vi "Sensor Interface.vi"(8 "error in (no error)":errorcluster) -> (0 "error out":errorcluster)   [LabVIEW 2020]
doc: "Sensor Interface thread"
uses:
  Controls/Sensor Interface.ctl
  FGV/Controls/FGV_State.ctl
  Controls/Data_Initialize.ctl
  Database/Controls/Account Database.ctl
  Controls/Events_User.ctl
  SubVIs/Message Queue/Enqueue Message (Single).vi
  <vilib>/Utility/error.llb/Error Cluster From Error Code.vi
  <vilib>/ErrorRing/Error Ring.xnode
  SubVIs/User Event - Stop/User Event - Stop.lvlib
  SubVIs/Message Queue/Message Queue.lvlib
panel:
  in  "Sensor Interface":T1
  # "[Covers: UI4]"
  # "[Covers: UI1]"
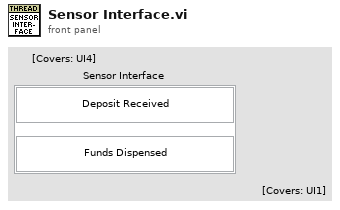
[diagram p1: front panel]
types:
  T1 = typedef "Sensor Interface.ctl" = cluster{"Deposit Received":bool, "Funds Dispensed":bool}
  T2 = enum32{"Invalid", "Standard", "Closed", "Hidden", "Minimized", "Maximized"}
  T3 = typedef "FGV_State.ctl" = enum16{"1 - OpenDatabase", "2 - Initialize Events", "3 - Initialize QMH", "4 - Close QMH", "5 - Close Events", "Read FGV", "Save Database", "Def"}
  T4 = typedef "FGV_Data.ctl" = cluster{"QMH":T5, "User Events":T6, "Database":T7[]}
  T5 = typedef "Message Queue.lvlib/All Message Queues.ctl" = cluster{"User Console":refnum<queue>, "Display Console":refnum<queue>, "Sensor Interface":refnum<queue>, "Process":refnum<queue>}
  T6 = typedef "Events_User.ctl" = cluster{"Stop User Console":refnum<user-event>, "Error User Console":refnum<user-event>, "Stop Sensor Interface ":refnum<user-event>, "Error Sensor Interface":refnum<user-event>}
  T7 = typedef "Account Database.ctl" = cluster{"Account Number":i32, "First Name":string, "Last Name":string, "Balance":dbl}
  T8 = typedef "Data_Initialize.ctl" = cluster{"Database":T7[], "User Events":T6}
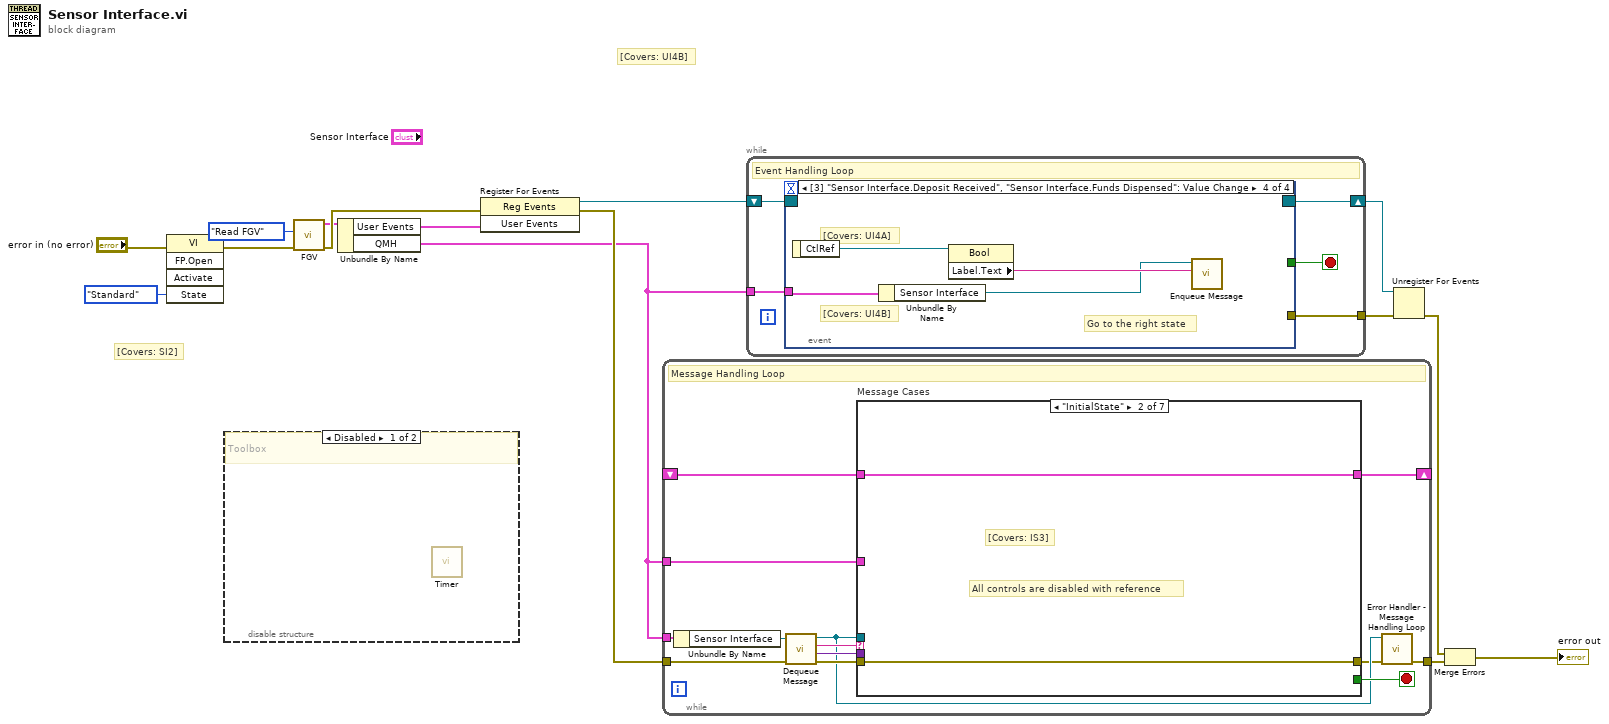
[diagram p0: block diagram]
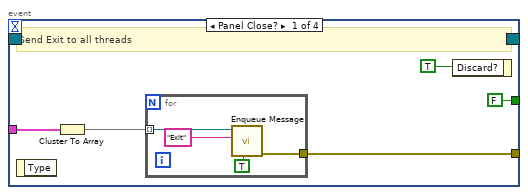
[diagram p3: hidden frame]
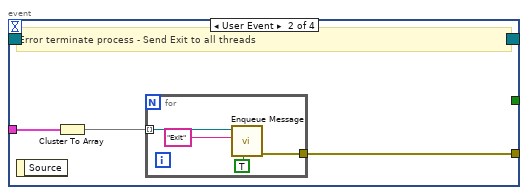
[diagram p4: hidden frame]
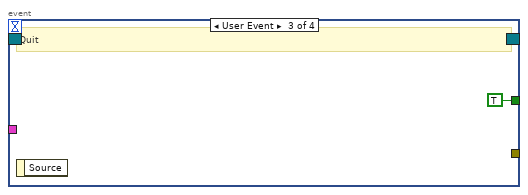
[diagram p5: hidden frame]
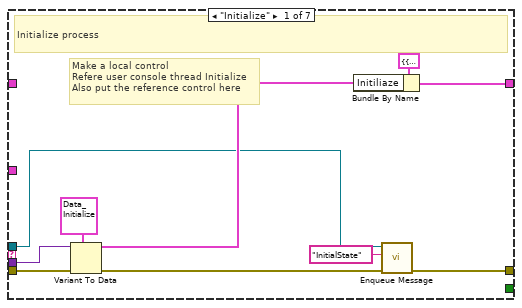
[diagram p6: hidden frame]
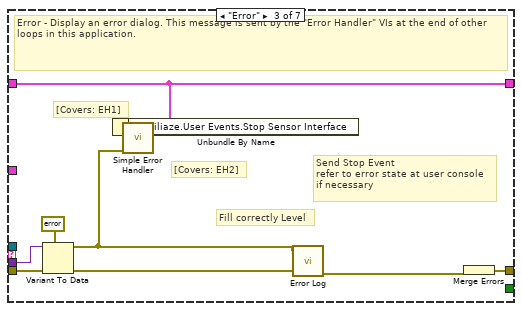
[diagram p7: hidden frame]
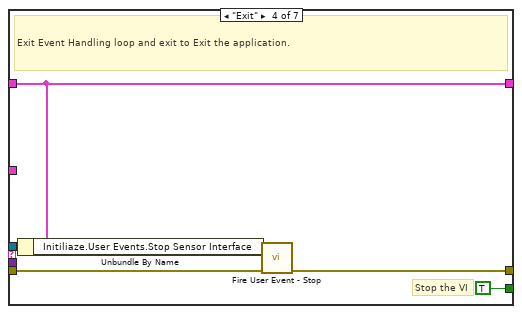
[diagram p8: hidden frame]
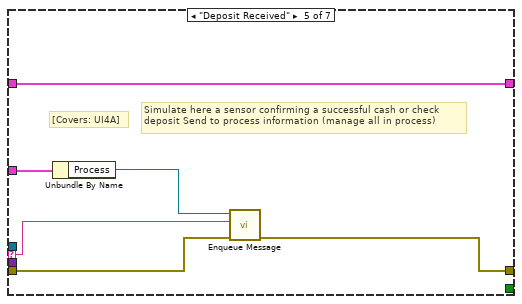
[diagram p9: hidden frame]
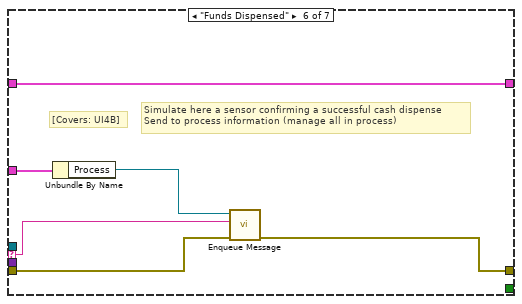
[diagram p10: hidden frame]
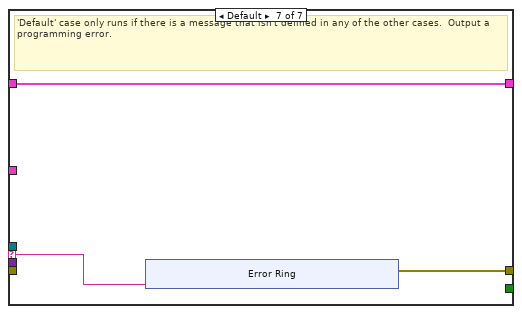
[diagram p11: hidden frame]
diagram:
  # "[Covers: UI4B]"
  # "[Covers: SI2]"
  n1 = invoke class="VI" method="FP.Open"(error in="error in (no error)", "State"=T2."Standard") -> (error out=w3:errorcluster)  [unwired: 3 in, 4 out]
  n2 = disable-structure shown="Disabled" {
    frame Disabled {
      # "Toolbox"
      n3 = call "Timer.vi"() -> ()  [unwired: 9 in, 3 out]
    }
    frame Enabled {
    }
  }
  n4 = call "FGV.vi"("error in (no error)"=w3, "FGV_State"=FGV_State."Read FGV") -> ("error out"=w13:errorcluster, "FGV 2"=w11:T4)  [unwired: 8 in]
  n5 = Unbundle By Name(w11) -> ("User Events"=w12:T6, "QMH"=w1:T5)
  n6 = register-events(error in=w13, w12) -> (reference out=w9:refnum<event-registration>, error out=w15:errorcluster)  [unwired: 1 in]
  n7 = while {
    tunnel: w1 -> [w18]
    shift-right: [w27] -> _
    shift-left: _ -> [w28]
    tunnel: w15 -> [w25]
    tunnel: [w20] -> w5
    tunnel: w1 -> [w16]
    stop <- w26 stop-if-true
    # "Message Handling Loop"
    n8 = Unbundle By Name(w18) -> ("Sensor Interface"=w17:refnum<queue>)
    n9 = call "Dequeue Message.vi"("error in (no error)"=w25, "Message Queue"=w17) -> ("error out"=w24:errorcluster, "Message Data"=w22:variant, "Message"=w23:string, "dup Message Queue"=w21:refnum<queue>)  [unwired: 6 in]
    n10 = case "Message Cases" shown="\"InitialState\"" w23 {
      selector: w23 -> [_ _ _ _ w56 w62 w66]
      tunnel: w21 -> [w32 _ _ _ _ _ _]
      tunnel: w24 -> [w36 w40 w48 w50 w55 w61 _]
      tunnel: [w30 w40 w45 w49 w54 w60 w67] -> w19
      tunnel: w28 -> [_ w39 w41 w52 w59 w65 w68]
      tunnel: [w38 w39 w41 w52 w59 w65 w68] -> w27
      tunnel: [_ _ _ TRUE _ _ _] -> w26
      tunnel: w22 -> [w33 _ w47 _ _ _ _]
      tunnel: w16 -> [_ _ _ _ w58 w64 _]
      frame "Initialize" {
        # "Make a local control\nRefere user console thread Initialize\nAlso put the reference control here"
        # "Initialize process"
        n11 = Variant To Data(error in=w36, type=T8 {"Database"=[], "User Events"={"Stop User Console"=refnum, "Error User Console"=refnum, "Stop Sensor Interface "=refnum, "Error Sensor Interface"=refnum}} ("Initiliaze"), Variant=w33) -> (data=w34:T8, error out=w31:errorcluster)
        n12 = Bundle By Name(cluster=cluster{"Initiliaze":T8} {"Initiliaze"={"Database"=[], "User Events"={"Stop User Console"=refnum, "Error User Console"=refnum, "Stop Sensor Interface "=refnum, "Error Sensor Interface"=refnum}}} ("Local Data"), "Initiliaze"=w34) -> (w38:cluster{"Initiliaze":T8})
        n13 = call-poly "Enqueue Message.vi"("error in (no error)"=w31, "Message"="InitialState", "Message Queue"=w32) -> ("error out"=w30:errorcluster)  [unwired: 7 in, 1 out]
      }
      frame "InitialState" {
        # "[Covers: IS3]"
        # "All controls are disabled with reference"
      }
      frame "Error" {
        # "Send Stop Event\nrefer to error state at user console \nif necessary"
        # "[Covers: EH2]"
        # "[Covers: EH1]"
        # "Fill correctly Level"
        # "Error - Display an error dialog. This message is sent by the \"Error Handler\" VIs at the end of other loops in this application."
        n14 = Variant To Data(error in=w48, type=errorcluster {"status"=FALSE, "code"=0, "source"=""} ("error constant"), Variant=w47) -> (data=w42:errorcluster, error out=w44:errorcluster)
        n15 = Unbundle By Name(w41) -> ()  [unwired: 1 out]
        n16 = call <vilib>:"Simple Error Handler.vi"("error in (no error)"=w42) -> ()  [unwired: 4 in, 5 out]
        n17 = call "Error Log.vi"("error in"=w44, "error happened"=w42) -> ("error out"=w43:errorcluster)  [unwired: 9 in]
        n18 = Merge Errors(w43) -> (w45:errorcluster)
      }
      frame "Exit" {
        # "Stop the VI"
        # "Exit Event Handling loop and exit to Exit the application."
        n19 = Unbundle By Name(w52) -> ("Initiliaze.User Events.Stop Sensor Interface"=w51:refnum<user-event>)
        n20 = call "Fire User Event - Stop.vi"("error in (no error)"=w50, "User Event - Stop"=w51) -> ("error out"=w49:errorcluster)  [unwired: 9 in]
      }
      frame "Deposit Received" {
        # "Simulate here a sensor confirming a successful cash or check\ndeposit Send to process information (manage all in process)"
        # "[Covers: UI4A]"
        n21 = Unbundle By Name(w58) -> ("Process"=w57:refnum<queue>)
        n22 = call-poly "Enqueue Message.vi"("error in (no error)"=w55, "Message"=w56, "Message Queue"=w57) -> ("error out"=w54:errorcluster)  [unwired: 7 in, 1 out]
      }
      frame "Funds Dispensed" {
        # "Simulate here a sensor confirming a successful cash dispense \nSend to process information (manage all in process)"
        # "[Covers: UI4B]"
        n23 = Unbundle By Name(w64) -> ("Process"=w63:refnum<queue>)
        n24 = call-poly "Enqueue Message.vi"("error in (no error)"=w61, "Message"=w62, "Message Queue"=w63) -> ("error out"=w60:errorcluster)  [unwired: 7 in, 1 out]
      }
      frame Default {
        # "'Default' case only runs if there is a message that isn't defined in any of the other cases.  Output a programming error."
        n25 = xnode "Error Ring"("parameter 0"=w66) -> ("error out"=w67:errorcluster)
      }
    }
    n26 = call "Error Handler - Message Handling Loop.vi"("error in (no error)"=w19, "Message Queue"=w21) -> ("dup error in"=w20:errorcluster)  [unwired: 8 in, 1 out]
  }
  n27 = while {
    tunnel: w1 -> [w80]
    shift-right: [w78] -> w7
    shift-left: w9 -> [w79]
    tunnel: [w76] -> w8
    stop <- w77 stop-if-true
    # "Event Handling Loop"
    n28 = event shown="[3] \"Sensor Interface.Deposit Received\", \"Sensor Interface.Funds Dispensed\": Value Change" {
      selector: w79 -> [_ _ _ _]
      dyn-events: [_ _ _ _] -> w78
      timeout: _ -> [_ _ _ _]
      tunnel: [FALSE ("Discard?") _ TRUE ("Discard?") _] -> w77
      tunnel: w80 -> [w84 w92 _ w98]
      tunnel: [w83 w91 _ _] -> w76
      event Panel Close? {
        # "Send Exit to all threads"
        n29 = event-data() -> ()  [unwired: 1 in, 1 out]
        n30 = Cluster To Array(cluster=w84) -> (array=w82:refnum<queue>[])
        n31 = for {
          tunnel: w82 -> [w89] mode=indexing
          tunnel: [w88] -> w83
          n32 = call-poly "Enqueue Message.vi"("Priority Message? (F)"=TRUE, "Message"="Exit", "Message Queue"=w89) -> ("error out"=w88:errorcluster)  [unwired: 7 in, 1 out]
        }
        n33 = event-data("Discard?"=TRUE) -> ()  [unwired: 1 in, 1 out]
      }
      event User Event {
        # "Error terminate process - Send Exit to all threads"
        n34 = event-data() -> ()  [unwired: 1 in, 1 out]
        n35 = Cluster To Array(cluster=w92) -> (array=w90:refnum<queue>[])
        n36 = for {
          tunnel: w90 -> [w96] mode=indexing
          tunnel: [w95] -> w91
          n37 = call-poly "Enqueue Message.vi"("Priority Message? (F)"=TRUE, "Message"="Exit", "Message Queue"=w96) -> ("error out"=w95:errorcluster)  [unwired: 7 in, 1 out]
        }
      }
      event User Event {
        # "Quit"
        n38 = event-data() -> ()  [unwired: 1 in, 1 out]
      }
      event Value Change {
        # "[Covers: UI4B]"
        # "Go to the right state"
        # "[Covers: UI4A]"
        n39 = event-data() -> ("CtlRef"=w99:refnum<vi>)  [unwired: 1 in]
        n40 = Unbundle By Name(w98) -> ("Sensor Interface"=w100:refnum<queue>)
        n41 = property class="Bool"(reference=w99) -> ("Label.Text"=w101:string)  [unwired: 1 in, 2 out]
        n42 = call-poly "Enqueue Message.vi"("Message"=w101, "Message Queue"=w100) -> ()  [unwired: 8 in, 2 out]
      }
    }
  }
  n43 = Unregister For Events(event registration refnum=w7, error in=w8) -> (error out=w6:errorcluster)
  n44 = Merge Errors(w6, w5) -> (→"error out":errorcluster)
